vi "BIO_set_recv_timeout.vi"(8 "error in (no error)":errorcluster, 10 "RECV timeout (ms)":u32=10000, 11 "BIO in":refnum<class "BIO.lvclass">) -> (0 "error out":errorcluster, 3 "BIO out":refnum<class "BIO.lvclass">)   [LabVIEW 2013, in "SSL_Lib.lvlib" / "BIO.lvclass"]
uses:
  BIO.lvclass
  SSL-Lib/SSL-Lib.lvclass
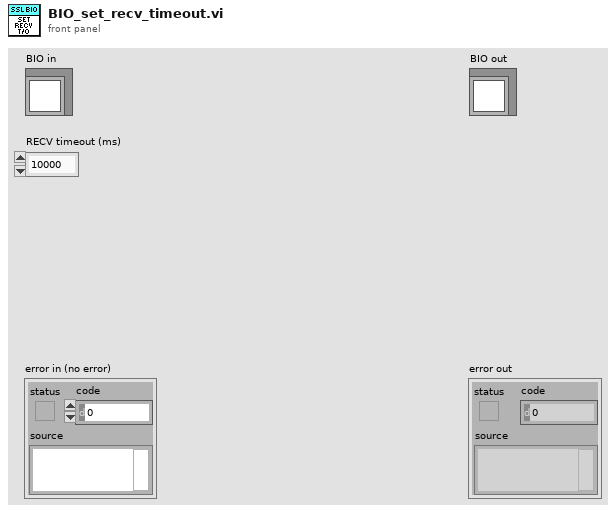
[diagram p1: front panel]
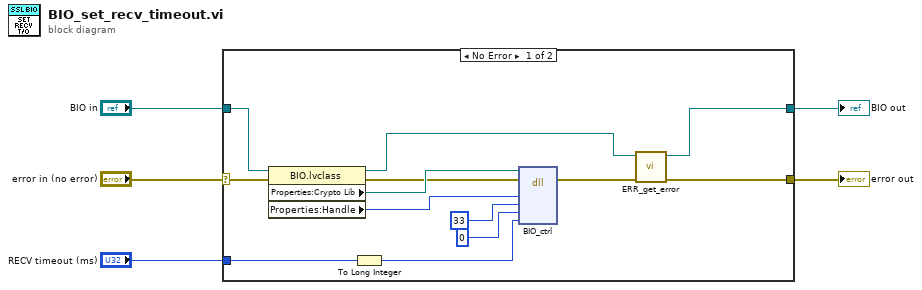
[diagram p0: block diagram]
diagram:
  n1 = case shown="No Error" "error in (no error)" {
    selector: "error in (no error)" -> [w15 w20]
    tunnel: [w9 w20] -> w4
    tunnel: [w7 w19] -> w2
    tunnel: "BIO in" -> [w14 w19]
    tunnel: "RECV timeout (ms)" -> [w16 _]
    frame No Error {
      n2 = property class="BIO.lvclass"(reference=w14, error in=w15) -> (reference out=w8:refnum<class "BIO.lvclass">, error out=w11:errorcluster, "Properties:Crypto Lib"=w12:path, "Properties:Handle"=w13:u64)
      n3 = To Long Integer(number=w16) -> (32bit integer=w6:i32)
      n4 = dll-call lib="C:/Program Files (x86)/National Instruments/Shared/nissl/NIlibeay32.dll" fn="BIO_ctrl"(path in=w12, error in=w11, "BIO"=w13, "cmd"=33, "larg"=0, "parg"=w6) -> (error out=w10:errorcluster)  [unwired: 6 in, 1 out]
      n5 = call "ERR_get_error.vi"("error in (no error)"=w10, "SSL-Lib in"=w8) -> ("error out"=w9:errorcluster, "SSL-Lib out"=w7:refnum<class "BIO.lvclass">)  [unwired: 8 in]
    }
    frame Error {
    }
  }
  "error out" <- w4
  "BIO out" <- w2
